vi "ConfigureMarkerSearch.vi"(8 "error in (no error)":errorcluster, 11 "Keysight44xx in":refnum<class "Keysight44xx.lvclass">) -> (0 "error out":errorcluster, 3 "Keysight44xx out":refnum<class "Keysight44xx.lvclass">)   [LabVIEW 2018, in "SpecAnPlugins.lvlib" / "Keysight44xx.lvclass"]
doc: "This VI configures the marker peak excursion and marker threshold values. The marker peak excursion specifies the minimum amplitude variation that can be recognized as a peak or minimum by the marker. The marker threshold specifies a lower bound for ALL marker search VIs."
uses:
  Keysight44xx.lvclass
  C:/Users/ico/Documents/Projects/NistPluggableModules/SpecAn/SpecAnPlugins/SpecAnBaseClass/SpecAnBase.lvclass
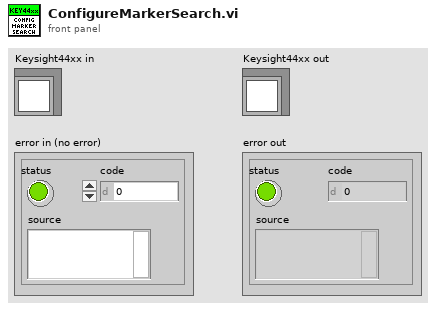
[diagram p1: front panel]
types:
  T1 = typedef "SpecAnPlugins.lvlib/SpecAnBase.lvclass/Acquisition.ctl" = cluster{"Handle":string, "Connected":bool, "Enabled":bool, "SweepModeContinuous":bool, "NumberOfSweeps":i32, "DetectorTypeAuto":bool, "DetectorType":i32, "VerticalScale":i32, "MaximumTime(seconds)":dbl}
  T2 = typedef "SpecAnPlugins.lvlib/SpecAnBase.lvclass/Markers.ctl" = cluster{"MarkerEnabled":bool, "MarkerThreshold":dbl, "PeakExcursion":dbl, "SignalTrackEnabled":bool, "MarkerPosition":dbl, "Instrument Setting (Frequency Center)":i32, "Marker search (Minimum)":i32, "ActiveMarker":string, "MarkerFrequencyCounter":bool, "FrequencyCounterResolution":dbl}
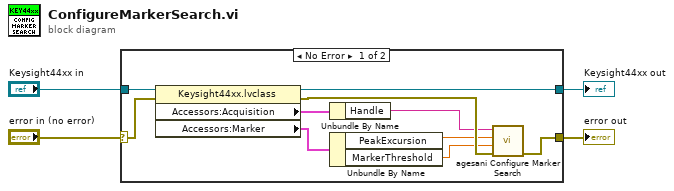
[diagram p0: block diagram]
diagram:
  n1 = case shown="No Error" "error in (no error)" {
    selector: "error in (no error)" -> [w13 w16]
    tunnel: [w8 w16] -> w3
    tunnel: "Keysight44xx in" -> [w14 w15]
    tunnel: [w12 w15] -> w1
    frame No Error {
      n2 = property class="Keysight44xx.lvclass"(reference=w14, error in=w13) -> (reference out=w12:refnum<class "Keysight44xx.lvclass">, error out=w9:errorcluster, "Accessors:Acquisition"=w11:T1, "Accessors:Marker"=w10:T2)
      n3 = Unbundle By Name(w11) -> ("Handle"=w7:string)
      n4 = Unbundle By Name(w10) -> ("PeakExcursion"=w6:dbl, "MarkerThreshold"=w5:dbl)
      n5 = call <instrlib>:"agesani Configure Marker Search.vi"("error in (no error)"=w9, "marker threshold (0.0)"=w5, "peak excursion (6.0)"=w6, "instrument handle"=w7) -> ("error out"=w8:errorcluster)  [unwired: 6 in, 1 out]
    }
    frame Error {
    }
  }
  "error out" <- w3
  "Keysight44xx out" <- w1
